vi "Configure AC Current.vi"(0 "VISA resource name":refnum<visa-resource-name>, 1 "NPLC":u16(ring) items=["0.00005", "1", "12", "15"], 5 "Auto Range? (T: Auto)":bool, 7 "Manual Range":dbl, 9 "Aperture Seconds":dbl, 11 "error in (no error)":errorcluster, 12 "Bandwidth (30)":u16(ring) items=["3", "30", "300"]) -> (4 "VISA resource name out":refnum<visa-resource-name>, 15 "error out":errorcluster)   [LabVIEW 2009, in "Keithley DMM7510.lvlib"]
doc: "This VI configures the AC Current measurement and the related parameters."
uses:
  Keithley DMM7510.lvlib
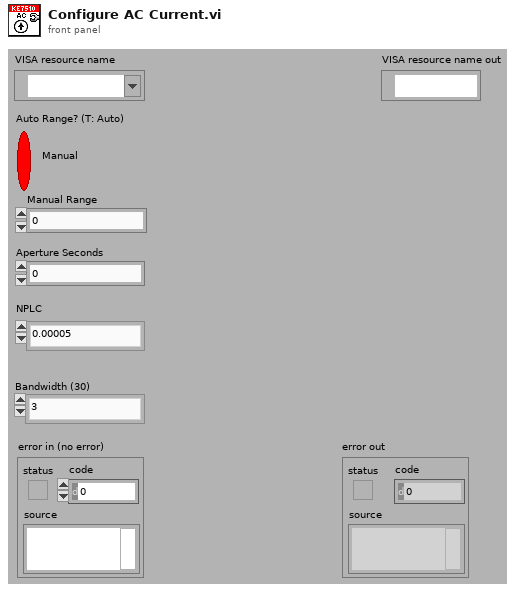
[diagram p1: front panel]
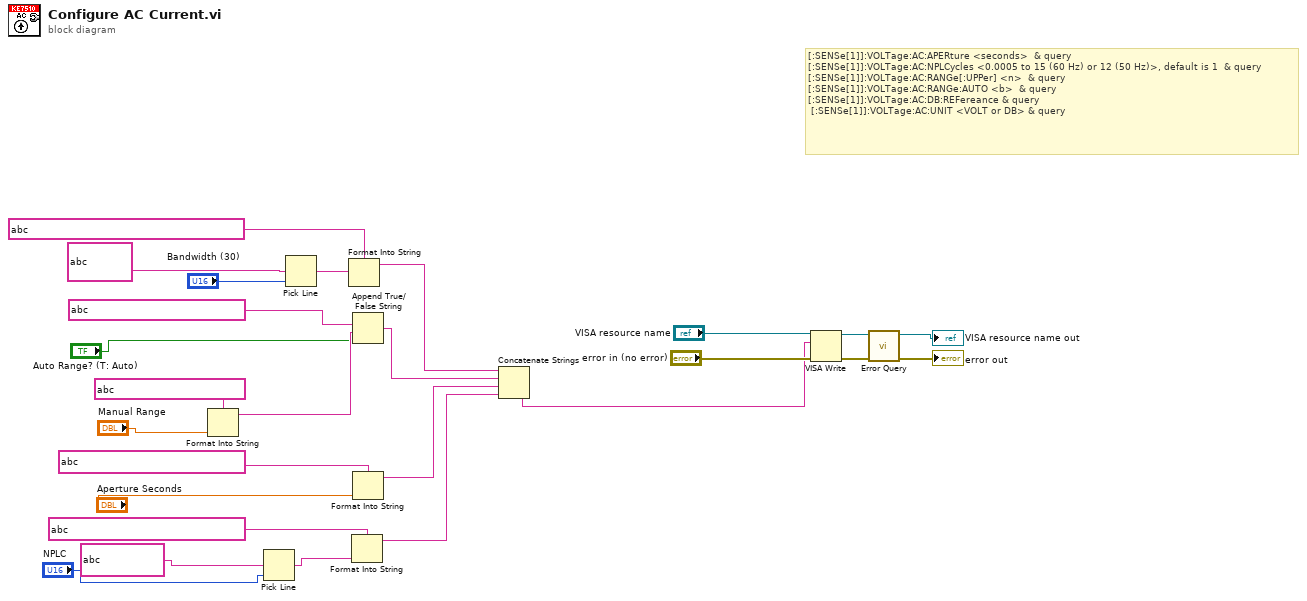
[diagram p0: block diagram]
diagram:
  # "[:SENSe[1]]:VOLTage:AC:APERture <seconds>  & query\n[:SENSe[1]]:VOLTage:AC:NPLCycles <0.0005 to 15 (60 Hz) or 12 (50 Hz)>, default is 1  & query\n[:SENSe[1]]:VOLTage:AC:RANGe[:UPPer] <n>  & query\n[:SENSe[1]]:VOLTage:AC:RANGe:AUTO <b>  & query\n[:SENSe[1]]:VOLTage:AC:DB:REFereance & query\n [:SENSe[1]]:VOLTage:AC:UNIT <VOLT or DB> & query"
  n1 = Format Into String(format string=string ?, "Manual Range") -> (resulting string=w21:string)  [unwired: 2 in, 1 out]
  n2 = Pick Line(multi-line string=string ?, line index="NPLC") -> (output string=w5:string)  [unwired: 1 in]
  n3 = Pick Line(multi-line string=string ?, line index="Bandwidth (30)") -> (output string=w8:string)  [unwired: 1 in]
  n4 = Format Into String(format string=string ?, w8) -> (resulting string=w18:string)  [unwired: 2 in, 1 out]
  n5 = Format Into String(format string=string ?, w5) -> (resulting string=w15:string)  [unwired: 2 in, 1 out]
  n6 = Append True/False String(1:"Auto Range? (T: Auto)", 2:w21, 3:string ?) -> (0:w17:string)  [unwired: 1 in]
  n7 = Format Into String(format string=string ?, "Aperture Seconds") -> (resulting string=w16:string)  [unwired: 2 in, 1 out]
  n8 = Concatenate Strings(w18, w17, w16, w15) -> (w14:string)
  n9 = VISA Write(VISA resource name="VISA resource name", write buffer=w14, error in (no error)="error in (no error)") -> (VISA resource name out=w13:refnum<visa-resource-name>, error out=w12:errorcluster)  [unwired: 1 out]
  n10 = call "Error Query.vi"("error in (no error)"=w12, "VISA resource name"=w13) -> ("error out"=→"error out":errorcluster, "VISA resource name out"=→"VISA resource name out":refnum<visa-resource-name>)  [unwired: 6 in, 2 out]
